vi "FRCts20_WebMethods_Application_GET.vi"(7 "httpRequestID":u32) -> ()   [LabVIEW 2014]
doc: "<B>GET</B> on the Application resource\n\nReturns application build revision and current competition.\n\nhttp://<server address>:<port>/FRCts/application"
uses:
  FRCts20_WebMethods.lvlib
  Backend/source/VI Source/FRCts20_Backend_API/FRCts20_Backend_API.lvlib
  Backend/source/VI Source/FRCts20_Backend_API/FRCts20_Backend_API_Application.vi
  Backend/source/VI Source/INI_Accessor/FRCts20_Backend_INI Controller.lvclass
  Backend/source/VI Source/FRCts20_Backend_API/FRCts20_Backend_API_Command_App.ctl
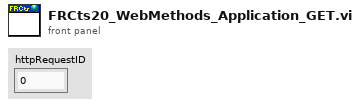
[diagram p1: front panel]
types:
  T1 = typedef "FRCts20_Backend_API.lvlib/FRCts20_Backend_API_Command_App.ctl" = string
  T2 = cluster{"Build Revision":string, "Current Competition":string}
  T3 = typedef "FRCts20_Backend_API.lvlib/FRCts20_Backend_API_Application.ctl" = cluster{"Revision":string, "APIReturn":string}
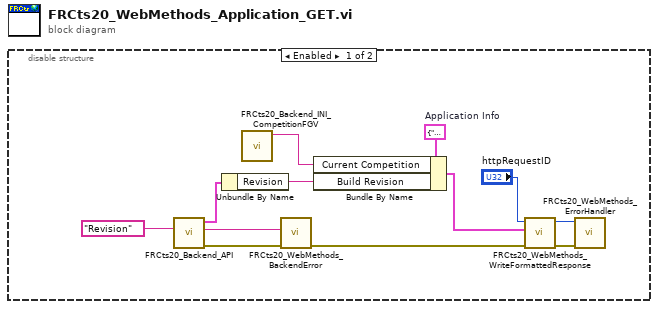
[diagram p0: block diagram]
diagram:
  n1 = disable-structure shown="Enabled" {
    frame Enabled {
      w9 = T2 {"Build Revision"="", "Current Competition"=""}  # Application Info
      n2 = call-poly "FRCts20_Backend_API.vi"("Command"=T1 "Revision") -> ("error out"=w11:errorcluster, "Status"=w10:string, "Application"=w12:T3)  [unwired: 8 in]
      n3 = Unbundle By Name(w12) -> ("Revision"=w8:string)
      n4 = call "FRCts20_Backend_INI_CompetitionFGV.vi"() -> ("Value out"=w7:string)  [unwired: 11 in]
      n5 = call "FRCts20_WebMethods_BackendError.vi"("error in (no error)"=w11, "Status"=w10) -> ("error out"=w6:errorcluster)  [unwired: 8 in, 1 out]
      n6 = Bundle By Name(cluster=w9, "Current Competition"=w7, "Build Revision"=w8) -> (w1:T2)
      n7 = call "FRCts20_WebMethods_WriteFormattedResponse.vi"("error in (no error)"=w6, "Response Cluster"=w1, "httpRequestID"="httpRequestID") -> ("error out"=w5:errorcluster, "httpRequestID out"=w4:u32)  [unwired: 7 in]
      n8 = call "FRCts20_WebMethods_ErrorHandler.vi"("error in"=w5, "httpRequestID"=w4) -> ()  [unwired: 9 in, 1 out]
    }
    frame Disabled {
    }
  }
